vi "Check Status.vi"(8 "error in (no error)":errorcluster, 11 "Lockin and Keithley Multimeter in":refnum<class "Lockin and Keithley Multimeter.lvclass">) -> (0 "error out":errorcluster, 1 "Status":string, 2 "Ready?":bool, 3 "Lockin and Keithley Multimeter out":refnum<class "Lockin and Keithley Multimeter.lvclass">)   [LabVIEW 2023, in "Lockin and Keithley Multimeter.lvclass"]
doc: "(Dynamic) Check if the instrument is powered on and update its member fields with the instrument's current status. Optionally return a text status message."
uses:
  Lockin and Keithley Multimeter.lvclass
  Lockin and Keithley Multimeter.lvclass/Lockin and Keithley Multimeter.ctl
  Utility Classes/Readable/Readable.lvclass
  Lockin/sr830/SR830.lvlib
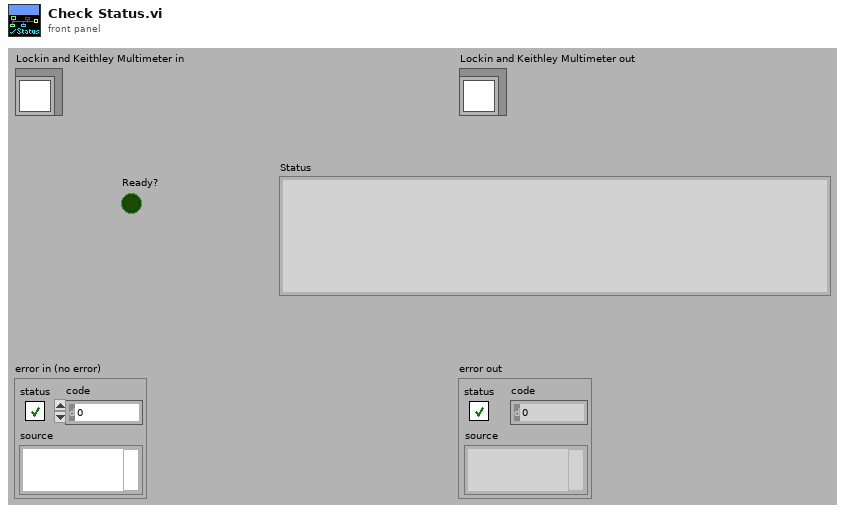
[diagram p1: front panel]
types:
  T1 = typedef "SR830.lvlib/Sensitivity_in_library.ctl" = u16
  T2 = cluster{"error":bool, "code":i32, "source":string}
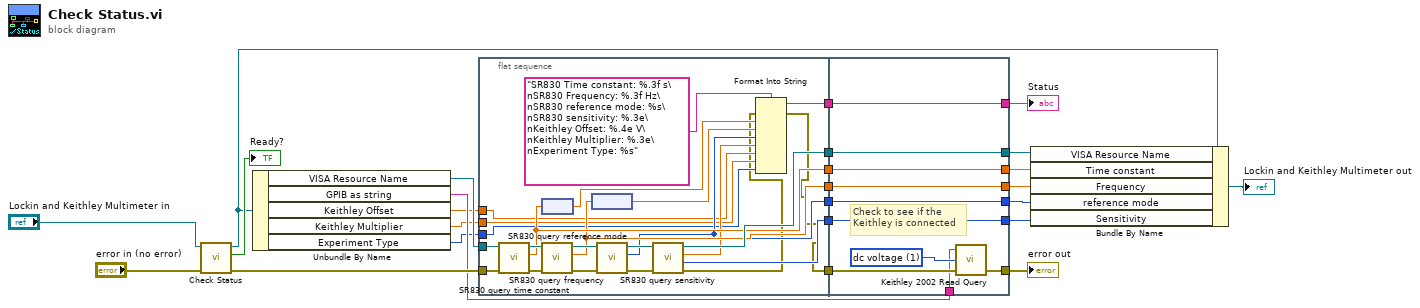
[diagram p0: block diagram]
diagram:
  n1 = call-parent "Check Status.vi"("error in (no error)"="error in (no error)", "Instrument in"="Lockin and Keithley Multimeter in") -> ("error out"=w22:errorcluster, "Ready?"=→"Ready?":bool, "Instrument out"=w21:refnum<class "Lockin and Keithley Multimeter.lvclass">)  [unwired: 6 in, 1 out]
  n2 = Unbundle By Name(w21) -> ("VISA Resource Name"=w14:refnum<visa-resource-name>, "GPIB as string"=w6:string, "Keithley Offset"=w4:dbl, "Keithley Multiplier"=w3:dbl, "Experiment Type"=w2:enum16{"CD", "EA", "None"})
  n3 = flat-sequence {
    tunnel: w14 -> [w42]
    tunnel: w22 -> [w41]
    tunnel: [w40] -> w13
    tunnel: [w26] -> w12
    tunnel: [w36] -> w11
    tunnel: [w35] -> w10
    tunnel: [w34] -> w9
    tunnel: [w33] -> w8
    tunnel: [w32] -> w7
    tunnel: w4 -> [w30]
    tunnel: w3 -> [w29]
    tunnel: w2 -> [w28]
    tunnel: [w53] -> w15
    tunnel: [w54] -> w16
    tunnel: [w55] -> w17
    tunnel: [w56] -> w18
    tunnel: [w57] -> w1
    tunnel: [w58] -> w19
    tunnel: w13 -> [w58]
    tunnel: w12 -> [w52]
    tunnel: w11 -> [w57]
    tunnel: w10 -> [w56]
    tunnel: w9 -> [w55]
    tunnel: w8 -> [w54]
    tunnel: w7 -> [w53]
    tunnel: w6 -> [w50]
    tunnel: [w49] -> w5
    frame #0 {
      n4 = call "SR830 query time constant.vi"("error in (no error)"=w41, "VISA resource name"=w42) -> ("error out"=w45:errorcluster, "time constant"=w35:dbl[unit], "VISA resource name out"=w43:refnum<visa-resource-name>)  [unwired: 7 in]
      n5 = node(w35) -> (w38:dbl)
      n6 = call "SR830 query frequency.vi"("error in (no error)"=w45, "VISA resource name"=w43) -> ("error out"=w46:errorcluster, "frequency"=w34:dbl[unit], "VISA resource name out"=w44:refnum<visa-resource-name>)  [unwired: 7 in]
      n7 = node(w34) -> (w37:dbl)
      n8 = call "SR830 query reference mode.vi"("error in (no error)"=w46, "VISA resource name"=w44) -> ("error out"=w48:errorcluster, "reference mode"=w33:enum16{"external", "internal"}, "VISA resource name out"=w47:refnum<visa-resource-name>)  [unwired: 7 in]
      n9 = call "SR830 query sensitivity.vi"("error in (no error)"=w48, "VISA resource name"=w47) -> ("error out"=w27:errorcluster, "Sensitivity"=w32:T1, "sensitivity"=w31:dbl[unit], "VISA resource name out"=w40:refnum<visa-resource-name>)  [unwired: 6 in]
      n10 = Format Into String(format string="SR830 Time constant: %.3f s\nSR830 Frequency: %.3f Hz\nSR830 reference mode: %s\nSR830 sensitivity: %.3e\nKeithley Offset: %.4e V\nKeithley Multiplier: %.3e\nExperiment Type: %s", error in=w27, w38, w37, w33, w31, w30, w29, w28) -> (resulting string=w36:string, error out=w26:errorcluster)  [unwired: 1 in]
    }
    frame #1 {
      w51 = u16 1 items=["ac voltage", "dc voltage", "2-wire resistance", "4-wire resistance", "ac current", "dc current", "frequency", "temperature"] ("function (Vdc:1)")
      # "Check to see if the \nKeithley is connected"
      n11 = call "Keithley 2002 Read Query.vi"("error in"=w52, "function (Vdc:1)"=w51, "GPIB Address"=w50) -> ("error out"=w49:T2)  [unwired: 1 in, 1 out]
    }
  }
  n12 = Bundle By Name(cluster=w21, "VISA Resource Name"=w19, "Time constant"=w18, "Frequency"=w17, "reference mode"=w16, "Sensitivity"=w15) -> (→"Lockin and Keithley Multimeter out":refnum<class "Lockin and Keithley Multimeter.lvclass">)
  "error out" <- w5
  "Status" <- w1
